vi "AR Drone - Simple NavData.vi"() -> ()   [LabVIEW 2014]
doc: "Very simple example showing how to use the base VIs to control the AR Drone and receive and display navigation data."
uses:
  <vilib>/LVH/AR Drone Toolkit/Decode NavData/Typedefs/NavData Demo.ctl
  <vilib>/LVH/AR Drone Toolkit/AR Drone.lvlib
panel:
  out "Battery Remaining":dbl(slide) scale=0.0..100.0
  out "NavData Out":T1
  in  "Control Cluster":T2 {"Yaw Speed" scale=-1.0..1.0; "Vertical Speed" scale=-1.0..1.0; "Pitch" scale=-1.0..1.0; "Roll" scale=-1.0..1.0}
  in  "stop":bool
  in  "Emergency Landing":bool
  in  "Take Off/Land":bool
  in  "Hover":bool
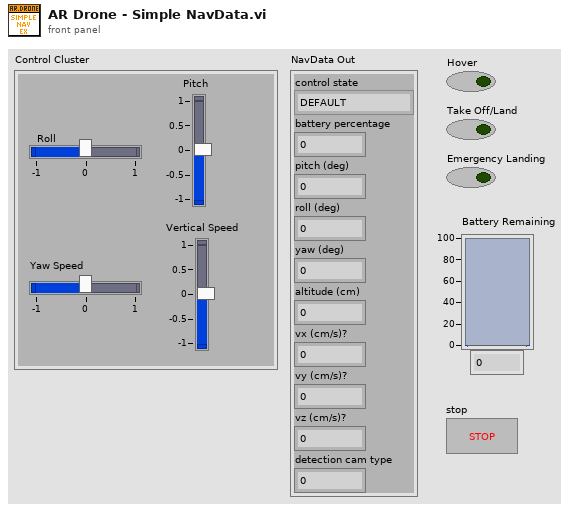
[diagram p1: front panel]
types:
  T1 = typedef "AR Drone.lvlib/NavData Demo.ctl" = cluster{"control state":enum32{"DEFAULT", "INIT", "LANDING", "FLYING", "HOVERING", "TEST", "TRANS_TAKEOFF", "TRANS_GOTOFIX", "TRANS_LANDING"}, "battery percentage":u32, "pitch (deg)":sgl, "roll (deg)":sgl, "yaw (deg)":sgl, "altitude (cm)":u32, "vx (cm/s)?":sgl, "vy (cm/s)?":sgl, "vz (cm/s)?":sgl, "detection cam type":u32}
  T2 = cluster{"Roll":sgl, "Pitch":sgl, "Vertical Speed":sgl, "Yaw Speed":sgl}
  T3 = typedef "AR Drone.lvlib/AR Drone Resource.ctl" = cluster{"UDP Control Connection":refnum<k16>, "UDP NavData Connection":refnum<k16>, "UDP Video Connection (Drone 1.0)":refnum<k16>, "TCP Video Connection (Drone 2.0)":refnum<k5>, "TCP Control Port Connection":refnum<k5>, "Drone IP address":string, "Drone Command Port":u16, "Drone NavData Port":u16, "Drone Vid Stream Port":u16, "Drone TCP Control Port":u16, "Home IP address":string, "Home Command Port":u16, "Home NavData Port":u16, "Home Vid Stream Port":u16, "Drone Version":i32}
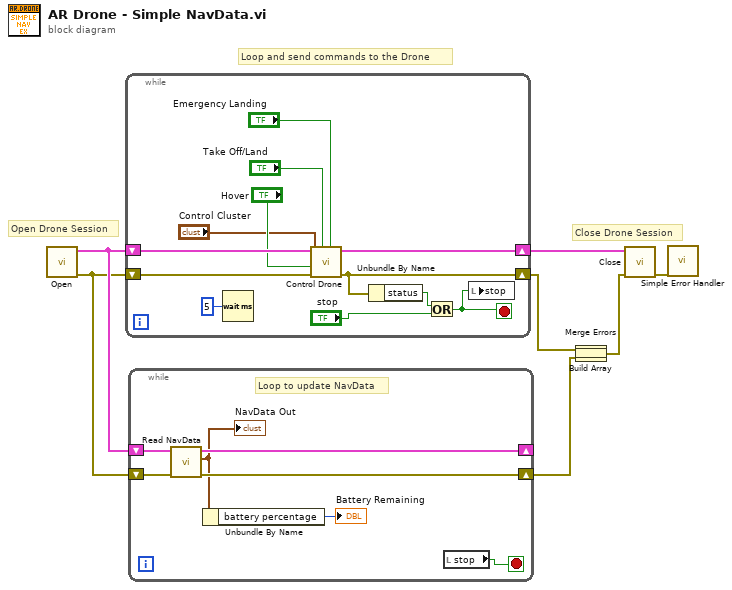
[diagram p0: block diagram]
diagram:
  # "Close Drone Session"
  # "Loop and send commands to the Drone"
  # "Open Drone Session"
  n1 = call <vilib>:"Open.vi"() -> ("error out"=w6:errorcluster, "AR Drone Resource"=w7:T3)  [unwired: 10 in]
  n2 = while {
    shift-right: [w15] -> w8
    shift-left: w7 -> [w19]
    shift-right: [w10] -> w4
    shift-left: w6 -> [w20]
    stop <- w9 stop-if-true
    n3 = Wait (ms)(milliseconds to wait=u32 5) -> ()  [unwired: 1 out]
    n4 = call <vilib>:"Control Drone.vi"("Emergency Landing"="Emergency Landing", "Takeoff/Land"="Take Off/Land", "error in (no error)"=w20, "Hover"="Hover", "Control Cluster"="Control Cluster", "AR Drone Resource"=w19) -> ("error out"=w10:errorcluster, "AR Drone Resource Out"=w15:T3)  [unwired: 4 in]
    n5 = Unbundle By Name(w10) -> ("status"=w12:bool)
    n6 = Or(x=w12, y="stop") -> (x .or. y?=w9:bool)
    n7 = local write "stop"(w9) -> ()
  }
  n8 = while {
    shift-right: [w25] -> _
    shift-left: w7 -> [w26]
    shift-right: [w23] -> w5
    shift-left: w6 -> [w24]
    stop <- w27 stop-if-true
    # "Loop to update NavData"
    n9 = call <vilib>:"Read NavData.vi"("error in (no error)"=w24, "AR Drone Resource"=w26) -> ("error out"=w23:errorcluster, "NavData Out"=w22:T1, "AR Drone Resource Out"=w25:T3)  [unwired: 7 in]
    "NavData Out" <- w22
    n10 = Unbundle By Name(w22) -> ("battery percentage"=→"Battery Remaining":u32)
    n11 = local read "stop"() -> (w27:bool)
  }
  n12 = Build Array(w4, w5) -> (w1:errorcluster[])
  n13 = Merge Errors(w1) -> (w3:errorcluster)
  n14 = call <vilib>:"Close.vi"("error in (no error)"=w3, "AR Drone Resource"=w8) -> ("error out"=w2:errorcluster)  [unwired: 9 in]
  n15 = call <vilib>:"Simple Error Handler.vi"("error in (no error)"=w2) -> ()  [unwired: 4 in, 5 out]
